vi "Get Window Position.vi"(8 "error in (no error)":errorcluster, 11 "VI in":refnum<vi>) -> (0 "error out":errorcluster)   [LabVIEW 2014, in "Chart Module.lvlib"]
uses:
  Chart Module.lvlib
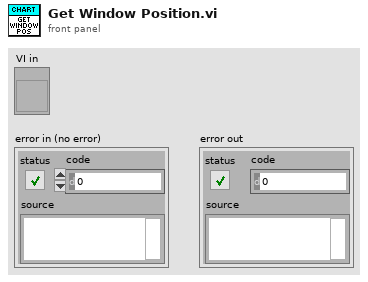
[diagram p1: front panel]
types:
  T1 = typedef "LVRectTypeDef.ctl" = cluster{"Left":i16, "Top":i16, "Right":i16, "Bottom":i16}
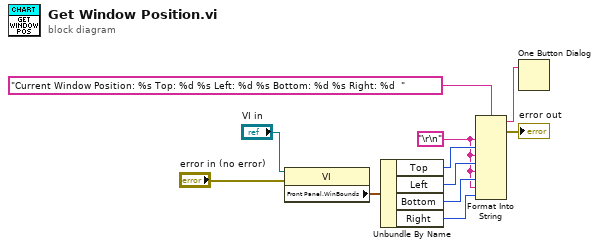
[diagram p0: block diagram]
diagram:
  w2 = "\r\n"
  n1 = property class="VI"(reference="VI in", error in="error in (no error)") -> ("Front Panel.WinBounds"=w11:T1)  [unwired: 2 out]
  n2 = Unbundle By Name(w11) -> ("Top"=w6:i16, "Left"=w5:i16, "Bottom"=w3:i16, "Right"=w1:i16)
  n3 = Format Into String(format string="Current Window Position: %s Top: %d %s Left: %d %s Bottom: %d %s Right: %d  ", w2, w6, w2, w5, w2, w3, w2, w1) -> (resulting string=w9:string, error out=→"error out":errorcluster)  [unwired: 2 in]
  n4 = One Button Dialog(message=w9) -> ()  [unwired: 1 in, 1 out]
